vi "Load Components.vi"(8 "error in (no error)":errorcluster) -> (0 "error out":errorcluster, 3 "Components":refnum<class "Component.lvclass">[](array[class]))   [LabVIEW 2017, in "DSF System Explorer.lvlib"]
uses:
  DSF System Explorer.lvlib
  DSF Core.lvlibp/Classes/Component/Component.lvclass
  DSF Core.lvlibp/Classes/Component Loader/Component Loader.lvclass
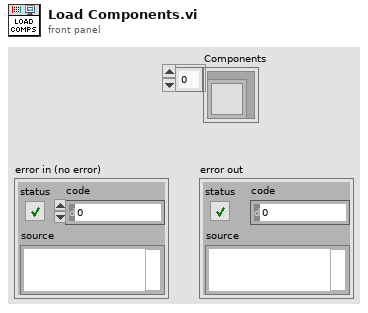
[diagram p1: front panel]
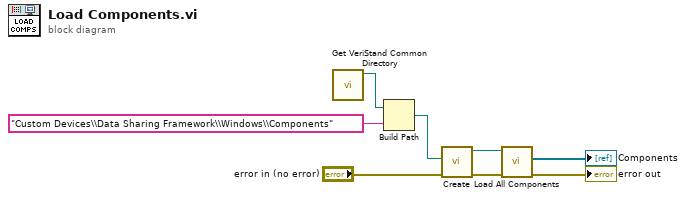
[diagram p0: block diagram]
diagram:
  n1 = call "Get VeriStand Common Directory.vi"() -> ("common directory"=w7:path)  [unwired: 11 in]
  n2 = Build Path(base path=w7, name or relative path="Custom Devices\\Data Sharing Framework\\Windows\\Components") -> (appended path=w5:path)
  n3 = call "Create.vi"("error in (no error)"="error in (no error)", "components directory"=w5) -> ("error out"=w3:errorcluster, "Component Loader out"=w4:refnum<class "Component Loader.lvclass">)  [unwired: 8 in]
  n4 = call "Load All Components.vi"("error in (no error)"=w3, "Component Loader in"=w4) -> ("error out"=→"error out":errorcluster, "Components"=→"Components":refnum<class "Component.lvclass">[])  [unwired: 7 in, 1 out]
